vi "Post Status from uService.vi"(8 "error in (no error)":errorcluster, 9 "payload":string, 10 "target":string, 11 "Father of all uServices in":refnum<class "Father of all uServices.lvclass">) -> (0 "error out":errorcluster, 3 "Father of all uServices out":refnum<class "Father of all uServices.lvclass">)   [LabVIEW 2026, in "TALOS.lvlib" / "Father of all uServices.lvlib" / "Father of all uServices.lvclass"]
doc: "This VI sends a JSON text to the Status Poster uService, which forwards the message to the Mattermost bot via an online API (HTTP Post). Mattermost bot performs status checks by comparing previously stored status to the newly arrived one."
uses:
  Father of all uServices.lvclass
  C:/LabVIEW Code/TALOS/builds/Actor Framework PPL/Actor Framework.lvlibp/1abvi3w/vi.lib/ActorFramework/Actor/Actor.lvclass
  Support VIs/Post.ctl
  Guardian/Guardian Messages/Message to uService Msg/Message to uService Msg.lvclass/Message to uService Msg.ctl
  Ancestor/Ancestor/Ancestor.lvclass/Ancestor.ctl
  Guardian/Guardian Messages/Message to uService Msg/Send Message to uService.vi
  Support VIs/Substitute Error.vi
  Support VIs/Generate Error.vi
  FGV/Error Memory/Get Error Description.vi
  Support VIs/Get PC name.vi
  Ancestor/Ancestor/Read ID.vi
  Support VIs/Get Class Name.vi
  FGV/Error Memory/Error Memory Core.vi
  <vilib>/AdvancedString/Delimited String to 1D String Array.vi
  <vilib>/AdvancedString/Delimited String to 1D String Array (string).vi
  Support VIs/Circus Root Path.vi
  FGV/Error Memory/Error Crt Lvl checker.vi
  FGV/Error Memory/Error Memory Core.vi/40c8088d-b597-4017-91af-faa98e00292e.vi
  FGV/Error Memory/Error Memory Core.vi/d4a3ab98-063c-4e44-b43d-fbdcfe6c2be2.vi
  builds/Actor Framework PPL/Actor Framework.lvlibp/1abvi3w/vi.lib/ActorFramework/Actor/Read Caller Enqueuer.vi
  builds/Actor Framework PPL/Actor Framework.lvlibp/1abvi3w/vi.lib/ActorFramework/Message Enqueuer/Enqueue.vi
  Support VIs/Global Memory.vi
  <vilib>/Utility/LVClass/Get LV Class Name.vi
  Support VIs/Is in Packed Library.vi
  Support VIs/TALOS Root path.vi
  Support VIs/Read CSV worksheet.vi
  Support VIs/Global Constants.vi
  <vilib>/Utility/error.llb/General Error Handler.vi
  Support VIs/Error Log.vi
  Guardian/Guardian Messages/Message to uService Msg/Message to uService Msg.lvclass
  Ancestor/Ancestor/Ancestor.lvclass
  <vilib>/Comparison/Equal/Equal Functor/Equal Functor.lvclass
  TALOS.lvlib
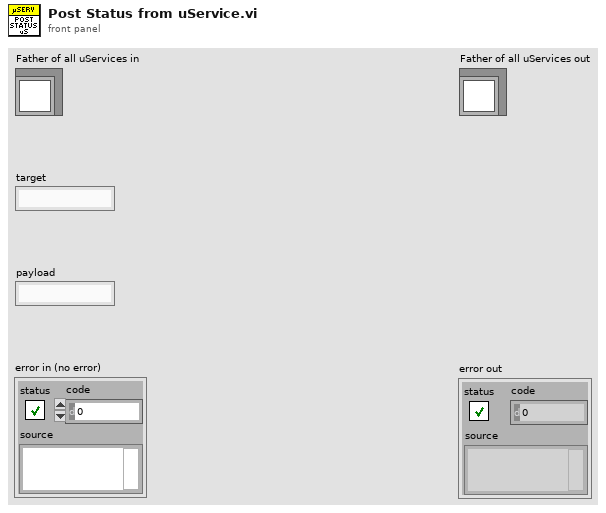
[diagram p1: front panel]
types:
  T1 = typedef "TALOS.lvlib/Post.ctl" = cluster{"target":string, "payload":string}
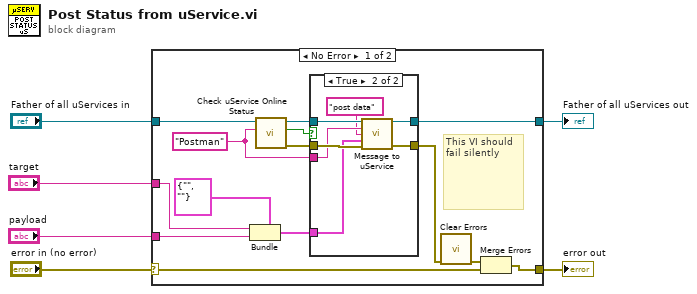
[diagram p0: block diagram]
diagram:
  n1 = case shown="No Error" "error in (no error)" {
    selector: "error in (no error)" -> [w15 w31]
    tunnel: [w13 w31] -> w5
    tunnel: [w20 w30] -> w3
    tunnel: "Father of all uServices in" -> [w11 w30]
    tunnel: "payload" -> [w19 _]
    tunnel: "target" -> [w18 _]
    frame No Error {
      w9 = "Postman"
      # "This VI should fail silently"
      n2 = Bundle(cluster=T1 {"target"="", "payload"=""} ("post"), "target"=w18, "payload"=w19) -> (w17:T1)
      n3 = call "Check uService Online Status.vi"("String"=w9, "Father of all uServices in"=w11) -> ("error out"=w8:errorcluster, "uService online?"=w7:bool, "Father of all uServices out"=w10:refnum<class "Father of all uServices.lvclass">)  [unwired: 7 in]
      n4 = case shown="True" w7 {
        tunnel: w10 -> [w22 w28]
        tunnel: [w22 w27] -> w20
        tunnel: w9 -> [_ w26]
        tunnel: w17 -> [_ w24]
        tunnel: [w21 w23] -> w16
        tunnel: w8 -> [w21 w29]
        frame False {
        }
        frame True {
          n5 = call "Message to uService.vi"("Father of all uServices in"=w28, "uService ID"=w26, "Message"="post data", "Data"=w24, "error in (no error)"=w29) -> ("Father of all uServices out"=w27:refnum<class "Father of all uServices.lvclass">, "error out"=w23:errorcluster)  [unwired: 9 in]
        }
      }
      n6 = call <vilib>:"Clear Errors.vi"("error in (no error)"=w16) -> ("error out"=w14:errorcluster)  [unwired: 5 in, 1 out]
      n7 = Merge Errors(w14, w15) -> (w13:errorcluster)
    }
    frame Error {
    }
  }
  "error out" <- w5
  "Father of all uServices out" <- w3
